vi "Get Name.vi"(8 "error in (no error)":errorcluster, 11 "Dependency Source in":refnum<class "Dependency Source_VIPM.lvclass">) -> (0 "error out":errorcluster, 2 "Dependency Source Name":string, 3 "Dependency Source out":refnum<class "Dependency Source_VIPM.lvclass">)   [LabVIEW 2019, in "Project.Dependencies Finder.lvlib" / "Dependency Source_VIPM.lvclass"]
doc: "Return the name of the dependency source. \n\nThis implementation returns 'VIPM'."
uses:
  Dependency Source_VIPM.lvclass
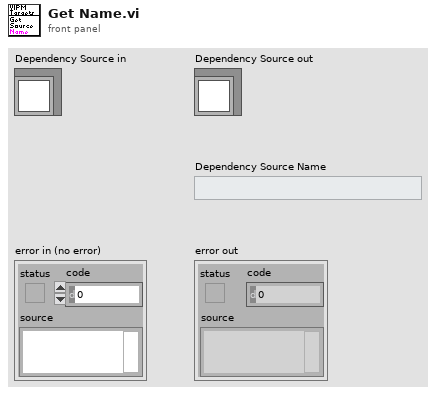
[diagram p1: front panel]
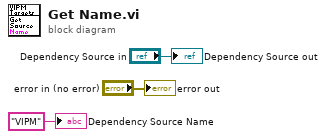
[diagram p0: block diagram]
diagram:
  "error out" <- "error in (no error)"
  "Dependency Source Name" <- "VIPM" ("Dependency Source Name")
  "Dependency Source out" <- "Dependency Source in"
